vi "Rabi Pulse 3.vi"() -> ()   [LabVIEW 2012]
uses:
  <vilib>/DAQmx/read.llb/DAQmx Read (Digital Bool 1Line 1Point).vi
  <vilib>/DAQmx/create/channels.llb/DAQmx Create Channel (DI-Digital Input).vi
  <vilib>/Utility/file.llb/Write To Spreadsheet File (DBL).vi
  <vilib>/DAQmx/miscellaneous.llb/DAQmx Fill In Error Info.vi
panel:
  in  "AOM Rest time":dbl
  in  "Signal delay":dbl
  in  "N Loop":i32=25000
  in  "APD signal width":dbl
  out "Run":bool
  out "size(s)":i32=225
  in  "file path (dialog if empty)":path=path "C:/Users/Ouyang Group/Documents/Data/12-5-13/Rabi pulse sequence 7"
  in  "AOM Pulse length":dbl=3e-07
  in  "Path to spinapi.dll":path=path "C:/SpinCore/SpinAPI/dll/spinapi64.dll"
  in  "stop":bool
  in  "start/restart":bool
  in  "MW width Max":dbl=5e-07
  in  "MW width step size":dbl=2e-09
  in  "MW width Min":dbl=5e-08
  in  "clock_freq (MHz)":dbl=300.0
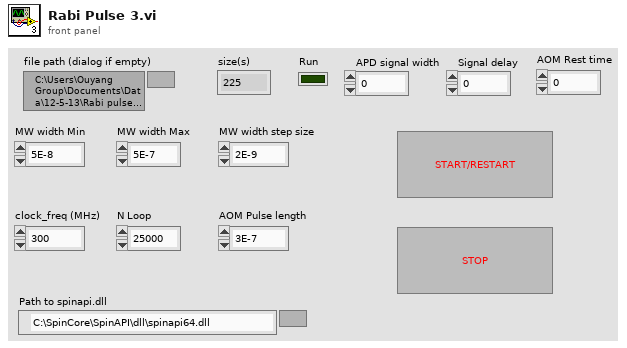
[diagram p1: front panel]
types:
  T1 = cluster{"Instruct Data":i32, "Op Code":i32, "Flags":bool[], "Comments":string, "Time (s)":dbl}[]
  T2 = cluster{"Instruct Data":i32, "Op Code":i32, "Flags":bool[], "Comments":string, "Time (s)":dbl}
  T3 = enum16{"Pulse Program", "Frequency Registers", "TX Phase Registers", "RX Phase Registers"}
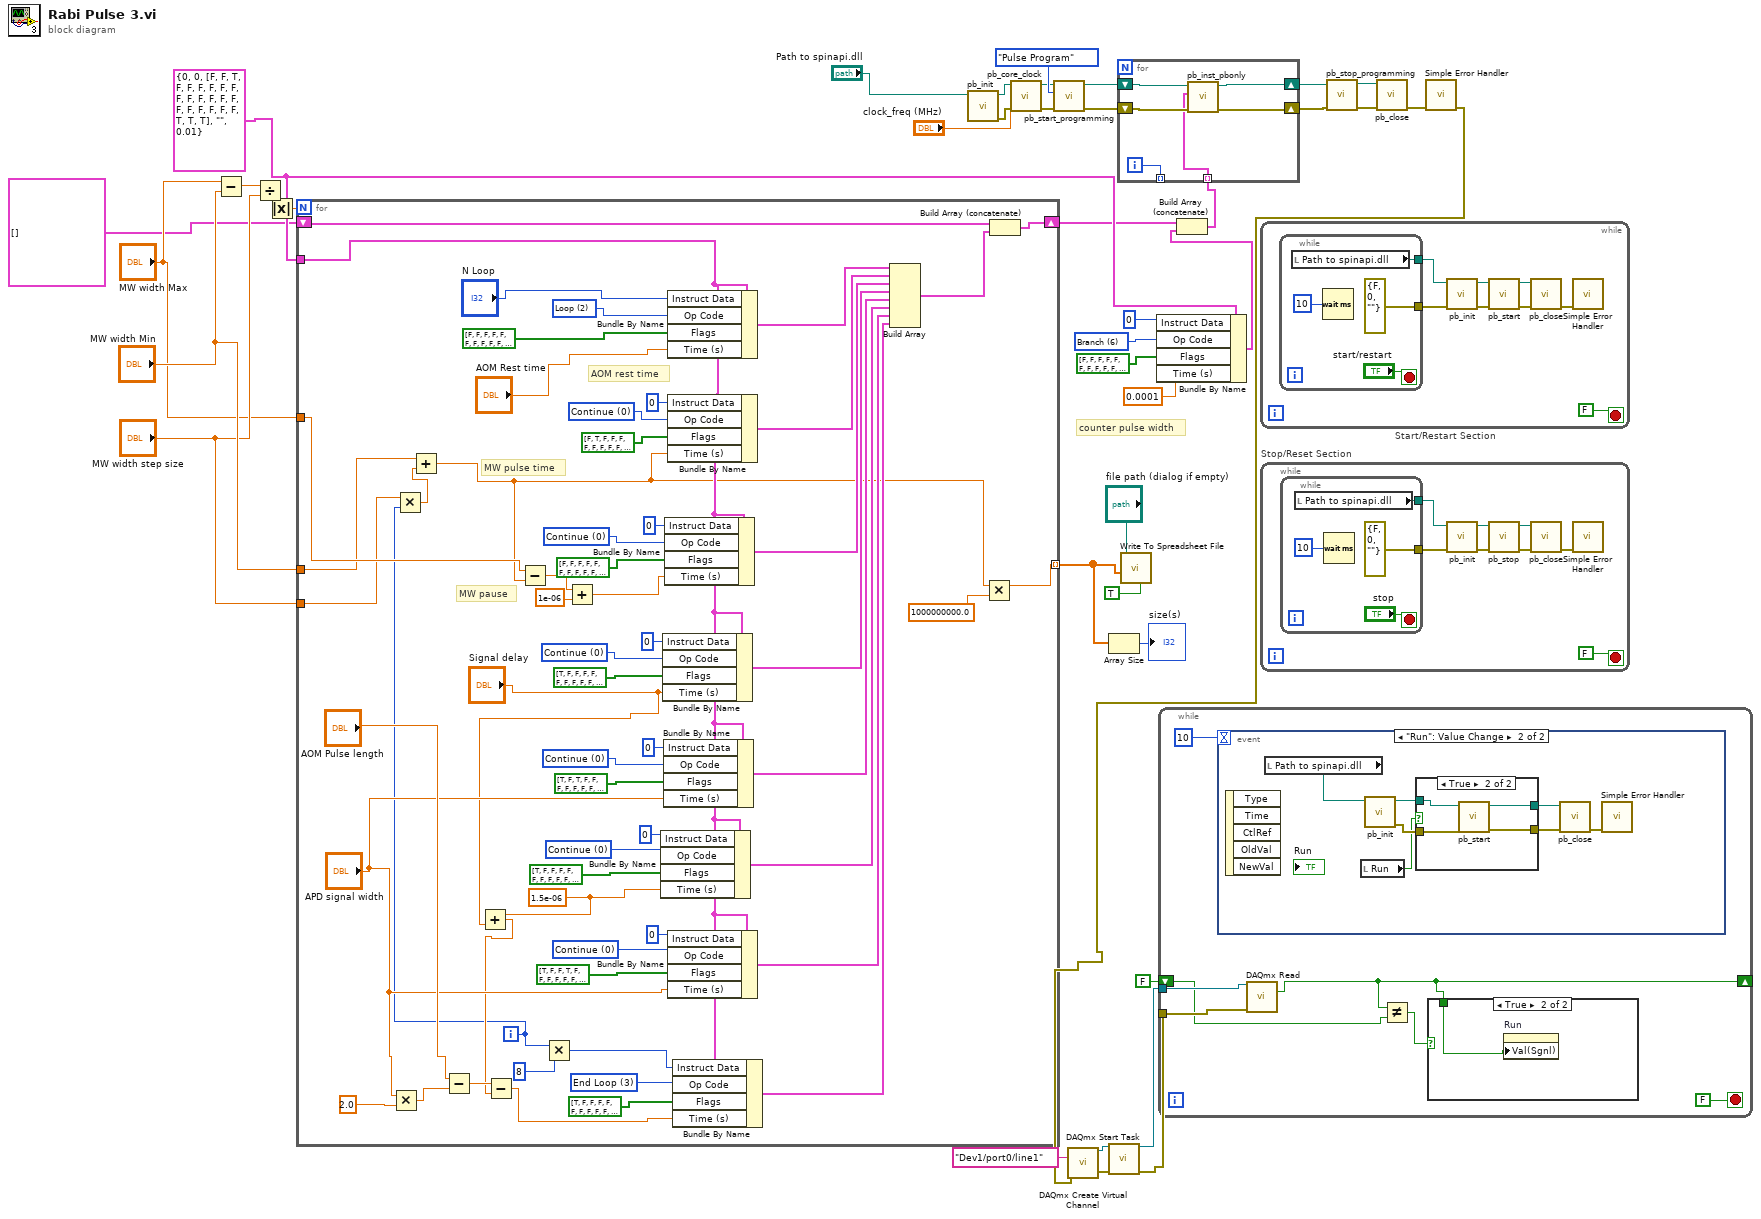
[diagram p0: block diagram]
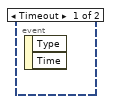
[diagram p2: hidden frame]
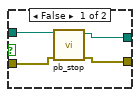
[diagram p3: hidden frame]
diagram:
  w7 = 6 items=["Continue", "Stop", "Loop", "End Loop", "JSR", "RTS", "Branch", "Long Delay", "Wait"] ("Op Code")
  w5 = T2 {"Instruct Data"=0, "Op Code"=0, "Flags"=[FALSE, FALSE, TRUE, FALSE, FALSE, FALSE, FALSE, FALSE, FALSE, FALSE, FALSE, FALSE, FALSE, FALSE, FALSE, FALSE, FALSE, FALSE, FALSE, FALSE, FALSE, TRUE, TRUE, TRUE], "Comments"="", "Time (s)"=0.01} ("PB Inst 2")
  # "counter pulse width"
  n1 = Subtract(x="MW width Max", y="MW width Min") -> (x-y=w28:dbl)
  n2 = Divide(x=w28, y="MW width step size") -> (x/y=w27:dbl)
  n3 = Absolute Value(x=w27) -> (abs(x)=w10:dbl)
  n4 = for {
    N: w10 -> [_]
    tunnel: "MW width Min" -> [w44]
    tunnel: "MW width step size" -> [w45]
    tunnel: [w86] -> w20 mode=indexing
    tunnel: w5 -> [w65]
    shift-right: [w97] -> w3
    shift-left: T1 [] -> [w98]
    tunnel: "MW width Max" -> [w52]
    i -> [w46]
    w54 = 0 items=["Continue", "Stop", "Loop", "End Loop", "JSR", "RTS", "Branch", "Long Delay", "Wait"] ("Op Code")
    w57 = 2 items=["Continue", "Stop", "Loop", "End Loop", "JSR", "RTS", "Branch", "Long Delay", "Wait"] ("Op Code")
    w67 = 0 items=["Continue", "Stop", "Loop", "End Loop", "JSR", "RTS", "Branch", "Long Delay", "Wait"] ("Op Code")
    w70 = 1.5e-06 ("Time (s)")
    w75 = 0 items=["Continue", "Stop", "Loop", "End Loop", "JSR", "RTS", "Branch", "Long Delay", "Wait"] ("Op Code")
    w81 = 3 items=["Continue", "Stop", "Loop", "End Loop", "JSR", "RTS", "Branch", "Long Delay", "Wait"] ("Op Code")
    w84 = 0 items=["Continue", "Stop", "Loop", "End Loop", "JSR", "RTS", "Branch", "Long Delay", "Wait"] ("Op Code")
    w92 = 0 items=["Continue", "Stop", "Loop", "End Loop", "JSR", "RTS", "Branch", "Long Delay", "Wait"] ("Op Code")
    w95 = 0 items=["Continue", "Stop", "Loop", "End Loop", "JSR", "RTS", "Branch", "Long Delay", "Wait"] ("Op Code")
    # "MW pause"
    # "AOM rest time"
    # "MW pulse time"
    n5 = Multiply(x="APD signal width", y=2.0) -> (x*y=w76:dbl)
    n6 = Multiply(x=w45, y=w46) -> (x*y=w47:dbl)
    n7 = Add(x=w44, y=w47) -> (x+y=w43:dbl)
    n8 = Subtract(x="AOM Pulse length", y=w76) -> (x-y=w71:dbl)
    n9 = Add(x=w70, y="Signal delay") -> (x+y=w59:dbl)
    n10 = Subtract(x=w71, y=w59) -> (x-y=w69:dbl)
    n11 = Subtract(x=w52, y=w43) -> (x-y=w51:dbl)
    n12 = Multiply(x=w46, y=8) -> (x*y=w48:i32)
    n13 = Add(x=w51, y=1e-06) -> (x+y=w49:dbl)
    n14 = Bundle By Name(cluster=w65, "Instruct Data"=0, "Op Code"=w84, "Flags"=bool[] [TRUE, FALSE, FALSE, FALSE, FALSE, FALSE, FALSE, FALSE, FALSE, FALSE, FALSE, FALSE, FALSE, FALSE, FALSE, FALSE, FALSE, FALSE, FALSE, FALSE, FALSE, TRUE, TRUE, TRUE], "Time (s)"=w70) -> (w60:T2)
    n15 = Bundle By Name(cluster=w65, "Instruct Data"=0, "Op Code"=w67, "Flags"=bool[] [TRUE, FALSE, FALSE, FALSE, FALSE, FALSE, FALSE, FALSE, FALSE, FALSE, FALSE, FALSE, FALSE, FALSE, FALSE, FALSE, FALSE, FALSE, FALSE, FALSE, FALSE, TRUE, TRUE, TRUE], "Time (s)"="Signal delay") -> (w63:T2)
    n16 = Bundle By Name(cluster=w65, "Instruct Data"=0, "Op Code"=w92, "Flags"=bool[] [TRUE, FALSE, TRUE, FALSE, FALSE, FALSE, FALSE, FALSE, FALSE, FALSE, FALSE, FALSE, FALSE, FALSE, FALSE, FALSE, FALSE, FALSE, FALSE, FALSE, FALSE, TRUE, TRUE, TRUE], "Time (s)"="APD signal width") -> (w64:T2)
    n17 = Bundle By Name(cluster=w65, "Instruct Data"=0, "Op Code"=w95, "Flags"=bool[] [FALSE, FALSE, FALSE, FALSE, FALSE, FALSE, FALSE, FALSE, FALSE, FALSE, FALSE, FALSE, FALSE, FALSE, FALSE, FALSE, FALSE, FALSE, FALSE, FALSE, FALSE, TRUE, TRUE, TRUE], "Time (s)"=w49) -> (w89:T2)
    n18 = Bundle By Name(cluster=w65, "Instruct Data"="N Loop", "Op Code"=w57, "Flags"=bool[] [FALSE, FALSE, FALSE, FALSE, FALSE, FALSE, FALSE, FALSE, FALSE, FALSE, FALSE, FALSE, FALSE, FALSE, FALSE, FALSE, FALSE, FALSE, FALSE, FALSE, FALSE, TRUE, TRUE, TRUE], "Time (s)"="AOM Rest time") -> (w91:T2)
    n19 = Bundle By Name(cluster=w65, "Instruct Data"=0, "Op Code"=w54, "Flags"=bool[] [FALSE, TRUE, FALSE, FALSE, FALSE, FALSE, FALSE, FALSE, FALSE, FALSE, FALSE, FALSE, FALSE, FALSE, FALSE, FALSE, FALSE, FALSE, FALSE, FALSE, FALSE, TRUE, TRUE, TRUE], "Time (s)"=w43) -> (w90:T2)
    n20 = Bundle By Name(cluster=w65, "Instruct Data"=0, "Op Code"=w75, "Flags"=bool[] [TRUE, FALSE, FALSE, TRUE, FALSE, FALSE, FALSE, FALSE, FALSE, FALSE, FALSE, FALSE, FALSE, FALSE, FALSE, FALSE, FALSE, FALSE, FALSE, FALSE, FALSE, TRUE, TRUE, TRUE], "Time (s)"="APD signal width") -> (w61:T2)
    n21 = Bundle By Name(cluster=w65, "Instruct Data"=w48, "Op Code"=w81, "Flags"=bool[] [TRUE, FALSE, FALSE, FALSE, FALSE, FALSE, FALSE, FALSE, FALSE, FALSE, FALSE, FALSE, FALSE, FALSE, FALSE, FALSE, FALSE, FALSE, FALSE, FALSE, FALSE, TRUE, TRUE, TRUE], "Time (s)"=w69) -> (w62:T2)
    n22 = Build Array(w91, w90, w89, w63, w64, w60, w61, w62) -> (w87:T1)
    n23 = Multiply(x=w43, y=1000000000.0) -> (x*y=w86:dbl)
    n24 = Build Array (concatenate)(w98, w87) -> (w97:T1)
  }
  n25 = call "pb_init.vi"("path in"="Path to spinapi.dll") -> ("error out"=w35:errorcluster, "path out"=w37:path)  [unwired: 3 in, 6 out]
  n26 = call "pb_core_clock.vi"("error in (no error)"=w35, "clock_freq (MHz)"="clock_freq (MHz)", "path in"=w37) -> ("error out"=w34:errorcluster, "path out"=w36:path)  [unwired: 7 in]
  n27 = call "pb_start_programming.vi"("error in (no error)"=w34, "Device"=T3."Pulse Program", "path in"=w36) -> ("error out"=w31:errorcluster, "path out"=w32:path)  [unwired: 1 in, 6 out]
  n28 = Array Size(array=w20) -> (size(s)=→"size(s)":i32)
  n29 = call-poly <vilib>:"Write To Spreadsheet File.vi"("transpose? (no:F)"=TRUE, "1D data"=w20, "file path (dialog if empty)"="file path (dialog if empty)") -> ()  [unwired: 5 in, 1 out]
  n30 = Bundle By Name(cluster=w5, "Instruct Data"=0, "Op Code"=w7, "Flags"=bool[] [FALSE, FALSE, FALSE, FALSE, FALSE, FALSE, FALSE, FALSE, FALSE, FALSE, FALSE, FALSE, FALSE, FALSE, FALSE, FALSE, FALSE, FALSE, FALSE, FALSE, FALSE, TRUE, TRUE, TRUE], "Time (s)"=0.0001) -> (w4:T2)
  n31 = Build Array (concatenate)(w3, w4) -> (w2:T1)
  n32 = for {
    shift-right: [w102] -> w30
    shift-left: w32 -> [w104]
    shift-right: [w101] -> w29
    shift-left: w31 -> [w103]
    tunnel: [w100] -> _ mode=indexing
    tunnel: w2 -> [w99] mode=indexing
    i -> [w100]
    n33 = call "pb_inst_pbonly.vi"("error in (no error)"=w103, "PB Instruction"=w99, "path in"=w104) -> ("error out"=w101:errorcluster, "path out"=w102:path)  [unwired: 2 in, 5 out]
  }
  n34 = while "Start/Restart Section" {
    stop <- FALSE stop-if-true
    n35 = while {
      tunnel: [errorcluster {"status"=FALSE, "code"=0, "source"=""} ("error in (no error)")] -> w109
      tunnel: [w113] -> w105
      stop <- "start/restart" stop-if-true
      n36 = local read "Path to spinapi.dll"() -> (w113:path)
      n37 = Wait (ms)(milliseconds to wait=u32 10) -> ()  [unwired: 1 out]
    }
    n38 = call "pb_init.vi"("error in (no error)"=w109, "path in"=w105) -> ("error out"=w108:errorcluster, "path out"=w111:path)  [unwired: 1 in, 7 out]
    n39 = call "pb_start.vi"("error in (no error)"=w108, "path in"=w111) -> ("error out"=w107:errorcluster, "path out"=w112:path)  [unwired: 1 in, 7 out]
    n40 = call "pb_close.vi"("error in (no error)"=w107, "path in"=w112) -> ("error out"=w106:errorcluster)  [unwired: 9 out]
    n41 = call <vilib>:"Simple Error Handler.vi"("error in (no error)"=w106) -> ()  [unwired: 1 in, 8 out]
  }
  n42 = while "Stop/Reset Section" {
    stop <- FALSE stop-if-true
    n43 = while {
      tunnel: [errorcluster {"status"=FALSE, "code"=0, "source"=""} ("error in (no error)")] -> w121
      tunnel: [w125] -> w117
      stop <- "stop" stop-if-true
      n44 = local read "Path to spinapi.dll"() -> (w125:path)
      n45 = Wait (ms)(milliseconds to wait=u32 10) -> ()  [unwired: 1 out]
    }
    n46 = call "pb_init.vi"("error in (no error)"=w121, "path in"=w117) -> ("error out"=w120:errorcluster, "path out"=w123:path)  [unwired: 1 in, 7 out]
    n47 = call "pb_stop.vi"("error in (no error)"=w120, "path in"=w123) -> ("error out"=w119:errorcluster, "path out"=w124:path)  [unwired: 8 out]
    n48 = call "pb_close.vi"("error in (no error)"=w119, "path in"=w124) -> ("error out"=w118:errorcluster)  [unwired: 9 out]
    n49 = call <vilib>:"Simple Error Handler.vi"("error in (no error)"=w118) -> ()  [unwired: 1 in, 8 out]
  }
  n50 = call "pb_stop_programming.vi"("error in (no error)"=w29, "path in"=w30) -> ("error out"=w38:errorcluster, "path out"=w39:path)  [unwired: 1 in, 7 out]
  n51 = call "pb_close.vi"("error in (no error)"=w38, "path in"=w39) -> ("error out"=w23:errorcluster)  [unwired: 9 out]
  n52 = call <vilib>:"Simple Error Handler.vi"("error in (no error)"=w23) -> ("error out"=w14:errorcluster)  [unwired: 1 in, 7 out]
  n53 = call-poly <vilib>:"DAQmx Create Virtual Channel.vi"("lines"=tag "Dev1/port0/line1", "error in"=w14) -> ("task out"=w12:refnum<k21>, "error out"=w11:errorcluster)  [unwired: 12 in]
  n54 = call <vilib>:"DAQmx Start Task.vi"("task/channels in"=w12, "error in"=w11) -> ("task out"=w13:refnum<k21>, "error out"=w16:errorcluster)  [unwired: 12 in]
  n55 = while {
    tunnel: w13 -> [w135]
    tunnel: w16 -> [w134]
    shift-right: [w131] -> _
    shift-left: FALSE ("data") -> [w133]
    stop <- FALSE stop-if-true
    n56 = event shown="[1] \"Run\": Value Change" {
      selector: _ -> [_ _]
      dyn-events: _ -> [_ _]
      timeout: 10 -> [_ _]
      event Timeout {
        n57 = event-data() -> ()  [unwired: 1 in, 2 out]
      }
      event "Run": Value Change {
        n58 = event-data() -> ()  [unwired: 1 in, 5 out]
        n59 = local read "Path to spinapi.dll"() -> (w136:path)
        n60 = local read "Run"() -> (w140:bool)
        n61 = call "pb_init.vi"("path in"=w136) -> ("error out"=w141:errorcluster, "path out"=w142:path)  [unwired: 2 in, 7 out]
        n62 = case shown="True" w140 {
          tunnel: w142 -> [w146 w150]
          tunnel: w141 -> [w145 w149]
          tunnel: [w144 w148] -> w138
          tunnel: [w143 w147] -> w137
          frame False {
            n63 = call "pb_stop.vi"("error in (no error)"=w145, "path in"=w146) -> ("error out"=w143:errorcluster, "path out"=w144:path)  [unwired: 8 out]
          }
          frame True {
            n64 = call "pb_start.vi"("error in (no error)"=w149, "path in"=w150) -> ("error out"=w147:errorcluster, "path out"=w148:path)  [unwired: 1 in, 7 out]
          }
        }
        n65 = call "pb_close.vi"("error in (no error)"=w137, "path in"=w138) -> ("error out"=w139:errorcluster)  [unwired: 9 out]
        n66 = call <vilib>:"Simple Error Handler.vi"("error in (no error)"=w139) -> ()  [unwired: 1 in, 8 out]
      }
    }
    n67 = call-poly <vilib>:"DAQmx Read.vi"("task/channels in"=w135, "error in"=w134) -> ("data"=w131:bool)  [unwired: 11 in, 2 out]
    n68 = Not Equal?(x=w131, y=w133) -> (x != y?=w132:bool)
    n69 = case shown="True" w132 {
      tunnel: w131 -> [_ w151]
      frame False {
      }
      frame True {
        n70 = property on="Run" class="Bool (strict)"("Val(Sgnl)"=w151) -> ()  [unwired: 2 in, 2 out]
      }
    }
  }
